vi "ep_Speed Estimation Check Data Vaild (1 Motor).vi"(0 "waveforms":waveform(dbl)[](array[waveform]), 2 "reset? (F)":bool, 5 "fundamental frequency [Hz]":dbl, 7 "speed estimation settings":cluster{"% overlap":dbl, "algorithm":T1}={"% overlap"=0.0, "algorithm"=enum."3-phase signals"}, 9 "nameplate information":T2, 11 "error in (no error)":errorcluster, 12 "window length [s]":dbl) -> (4 "signals":dbl[][](array[numeric]), 6 "spectra parameters":T3, 8 "dup speed estimation settings":cluster{"% overlap":dbl, "algorithm":T1}={"% overlap"=0.0, "algorithm"=enum."3-phase signals"}, 15 "error out":errorcluster)   [LabVIEW 2014, in "NI_EP_Motor Monitoring.lvlib"]
uses:
  <vilib>/addons/Electrical Power/Motor Monitoring/NI_EP_Motor Monitoring.lvlib
  <vilib>/addons/Electrical Power/Motor Monitoring/subVIs/ep_Demodulation Algorithm.ctl
  <vilib>/addons/Electrical Power/Power Measurement/NI_EP_Power Measurement.lvlib
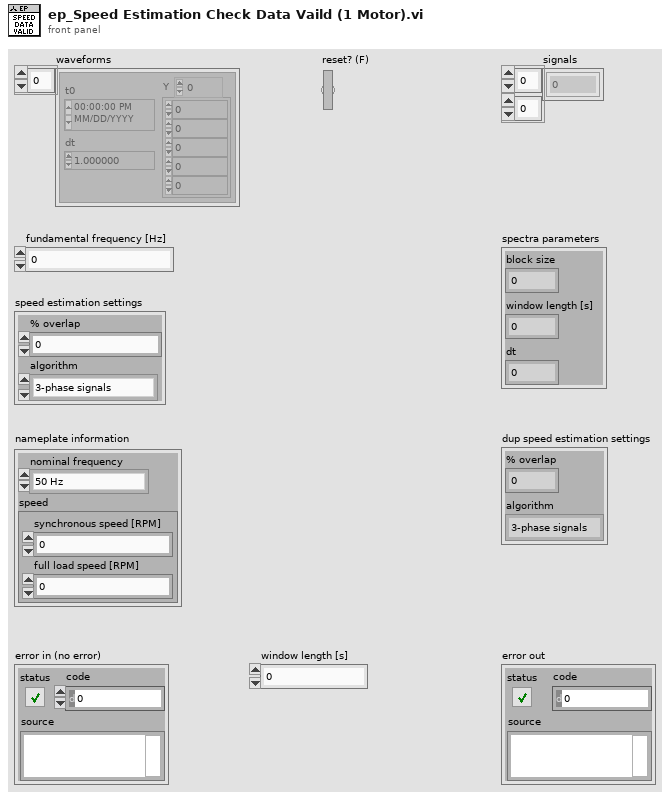
[diagram p1: front panel]
types:
  T1 = typedef "NI_EP_Motor Monitoring.lvlib/ep_Demodulation Algorithm.ctl" = enum16{"1-phase signal", "3-phase signals"}
  T2 = cluster{"nominal frequency":enum16{"50 Hz", "60 Hz"}, "speed":cluster{"synchronous speed [RPM]":dbl, "full load speed [RPM]":dbl}}
  T3 = cluster{"block size":i32, "window length [s]":dbl, "dt":dbl}
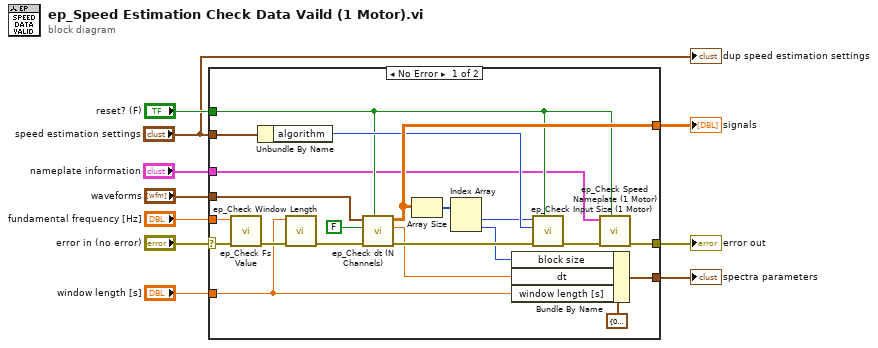
[diagram p0: block diagram]
diagram:
  n1 = case shown="No Error" "error in (no error)" {
    selector: "error in (no error)" -> [w23 w32]
    tunnel: "waveforms" -> [w30 _]
    tunnel: "reset? (F)" -> [w21 _]
    tunnel: "nameplate information" -> [w11 _]
    tunnel: "speed estimation settings" -> [w17 _]
    tunnel: [w28 _] -> w7
    tunnel: "window length [s]" -> [w12 _]
    tunnel: [w26 w32] -> w5
    tunnel: "fundamental frequency [Hz]" -> [w22 _]
    tunnel: [w19 _] -> w3
    frame No Error {
      n2 = call <vilib>:"ep_Check Fs Value.vi"("error in (no error)"=w23, "fundamental frequency [Hz]"=w22) -> ("error out"=w14:errorcluster)  [unwired: 9 in]
      n3 = Unbundle By Name(w17) -> ("algorithm"=w25:T1)
      n4 = call <vilib>:"ep_Check Window Length.vi"("error in (no error)"=w14, "window length [s]"=w12) -> ("error out"=w13:errorcluster)  [unwired: 9 in]
      n5 = call <vilib>:"ep_Check dt (N Channels).vi"("reset? (F)"=w21, "error in (no error)"=w13, "waveforms only? (F)"=FALSE, "waveforms"=w30) -> ("error out"=w18:errorcluster, "dt"=w15:dbl, "signals"=w28:dbl[][])  [unwired: 3 in, 2 out]
      n6 = Array Size(array=w28) -> (size(s)=w29:i32[])
      n7 = Index Array(array=w29) -> (element #1=w24:i32, element #2=w16:i32)  [unwired: 2 in]
      n8 = Bundle By Name(cluster=T3 {"block size"=0, "window length [s]"=0.0, "dt"=0.0}, "block size"=w16, "dt"=w15, "window length [s]"=w12) -> (w19:T3)
      n9 = call <vilib>:"ep_Check Input Size (1 Motor).vi"("check? (F)"=w21, "error in (no error)"=w18, "algorithm"=w25, "number of channels"=w24) -> ("error out"=w27:errorcluster)  [unwired: 7 in]
      n10 = call <vilib>:"ep_Check Speed Nameplate (1 Motor).vi"("check? (F)"=w21, "error in (no error)"=w27, "nameplate information"=w11) -> ("error out"=w26:errorcluster)  [unwired: 8 in]
    }
    frame Error {
    }
  }
  "error out" <- w5
  "signals" <- w7
  "spectra parameters" <- w3
  "dup speed estimation settings" <- "speed estimation settings"
